vi "distance limit.vi"(0 "Encoder Rate":dbl, 1 "Encoder Distance":dbl, 2 "Desired Rate":dbl, 3 "Forward Limit":dbl, 4 "Reverse Limit":dbl) -> (5 "Encoder Rate Out":dbl, 6 "Output Rate":dbl)   [LabVIEW 2012]
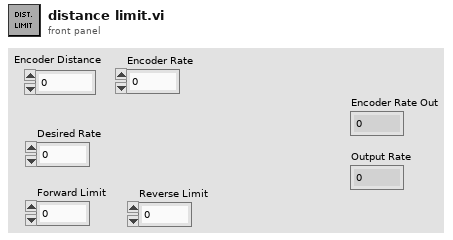
[diagram p1: front panel]
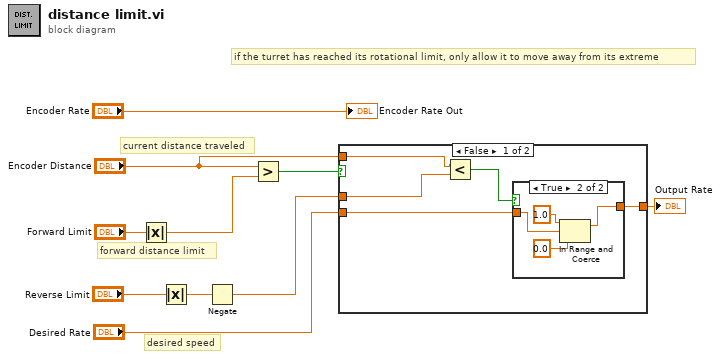
[diagram p0: block diagram]
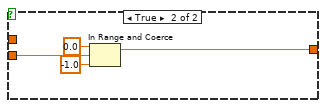
[diagram p3: hidden frame]
diagram:
  # "desired speed"
  # "forward distance limit"
  # "current distance traveled"
  # "if the turret has reached its rotational limit, only allow it to move away from its extreme"
  n1 = Absolute Value(x="Forward Limit") -> (abs(x)=w4:dbl)
  n2 = Absolute Value(x="Reverse Limit") -> (abs(x)=w2:dbl)
  n3 = Negate(x=w2) -> (-x=w1:dbl)
  n4 = Greater?(x="Encoder Distance", y=w4) -> (0:w9:bool)
  n5 = case shown="False" w9 {
    tunnel: "Desired Rate" -> [w13 w24]
    tunnel: "Encoder Distance" -> [w15 _]
    tunnel: [w12 w21] -> w5
    tunnel: w1 -> [w11 _]
    frame False {
      n6 = Less?(x=w15, y=w11) -> (x < y?=w14:bool)
      n7 = case shown="True" w14 {
        tunnel: w13 -> [w16 w18]
        tunnel: [w16 w17] -> w12
        frame False {
        }
        frame True {
          n8 = In Range and Coerce(upper limit=1.0, x=w18, lower limit=0.0) -> (coerced(x)=w17:dbl)  [unwired: 1 out]
        }
      }
    }
    frame True {
      n9 = In Range and Coerce(upper limit=0.0, x=w24, lower limit=-1.0) -> (coerced(x)=w21:dbl)  [unwired: 1 out]
    }
  }
  "Output Rate" <- w5
  "Encoder Rate Out" <- "Encoder Rate"
